vi "setExposureTime.vi"(0 "sCMOS cluster":cluster{"init":i16, "sCMOS handle":u32}, 1 "Exposure time (s)":dbl=0.009997714285714285) -> ()   [LabVIEW 2015]
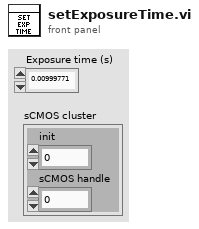
[diagram p1: front panel]
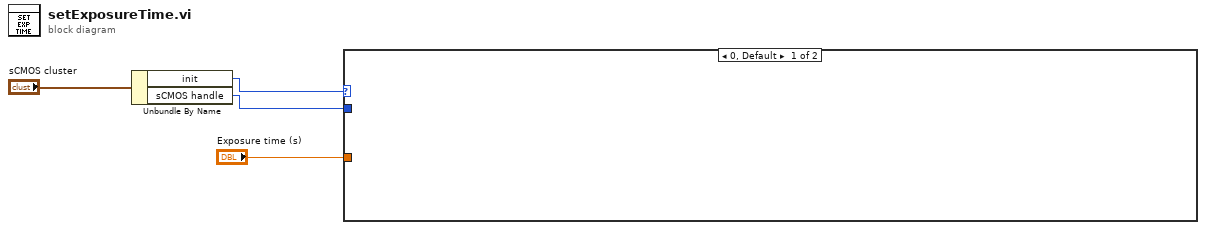
[diagram p0: block diagram]
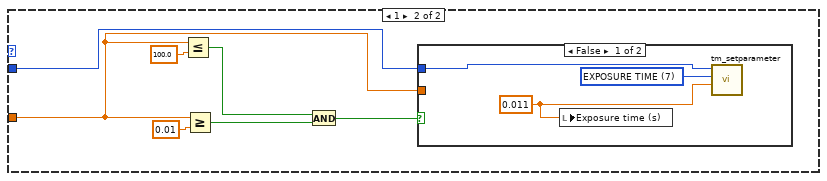
[diagram p2: hidden frame]
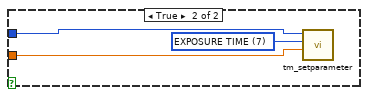
[diagram p3: hidden frame]
diagram:
  n1 = Unbundle By Name("sCMOS cluster") -> ("init"=w3:i16, "sCMOS handle"=w2:u32)
  n2 = case shown="0, Default" w3 {
    tunnel: "Exposure time (s)" -> [_ w5]
    tunnel: w2 -> [_ w11]
    frame 0, Default {
    }
    frame 1 {
      n3 = Less Or Equal?(x=w5, y=100.0 ("x")) -> (x <= y?=w8:bool)
      n4 = Greater Or Equal?(x=w5, y=0.01 ("x")) -> (x >= y?=w10:bool)
      n5 = And(x=w8, y=w10) -> (x .and. y?=w7:bool)
      n6 = case shown="False" w7 {
        tunnel: w11 -> [w14 w17]
        tunnel: w5 -> [_ w16]
        frame False {
          w12 = u32 7 items=["BINNING"=4215968, "BITS PER CHANNEL"=2, "ACTIVE VIEW INDEX"=3, "CCD MODE"=4, "SENSOR MODE"=5, "READOUT MODE"=6, "EXPOSURE TIME"=7, "CONTRAST GAIN"=8, "CONTRAST OFFSET"=9, "LIGHT MODE"=10, "SENSITIVITY"=11, "WHITE BALANCE"=12, "PHOTON IMAGING MODE"=13, "HIGH DYNAMIC RANGE MODE"=14, "TRIGGER SOURCE"=15, "TRIGGER ACTIVE"=16, "TRIGGER MODE"=17, "TRIGGER POLARITY"=18, "TRIGGER GLOBAL EXPOSURE"=19, "FIRST TRIGGER BEHAVIOR"=20, "TRIGGER TIMES"=21, "OUTPUT TRIGGER POLARITY"=22, "OUTPUT TRIGGER DELAY"=23, "OUTPUT TRIGGER PERIOD"=24, "TEMPERATURE"=25, "TEMPERATURE TARGET"=26, "SENSOR COOLER FAN"=27, "MECHANICAL SHUTTER"=28, "BACK FOCUS POSITION"=29, "FRAMEBUNDLE MODE"=30, "FRAMEBUNDLE NUMBER"=31, "LINEBUNDLE HEIGHT"=32, "TRIGGER CONNECTOR"=33, "IMAGE PIXEL TYPE"=34, "OUTPUT TRIGGER KIND"=35, "READOUT DIRECTION"=36, "CHANNEL SYNC"=37] ("Parameter")
          w13 = 0.011 ("Value in")
          n7 = local write "Exposure time (s)"(w13) -> ()
          n8 = call <userlib>:"tm_setparameter.vi"("Value in"=w13, "Parameter"=w12, "Handle in"=w14) -> ()  [unwired: 7 in, 2 out]
        }
        frame True {
          w15 = u32 7 items=["BINNING"=4215968, "BITS PER CHANNEL"=2, "ACTIVE VIEW INDEX"=3, "CCD MODE"=4, "SENSOR MODE"=5, "READOUT MODE"=6, "EXPOSURE TIME"=7, "CONTRAST GAIN"=8, "CONTRAST OFFSET"=9, "LIGHT MODE"=10, "SENSITIVITY"=11, "WHITE BALANCE"=12, "PHOTON IMAGING MODE"=13, "HIGH DYNAMIC RANGE MODE"=14, "TRIGGER SOURCE"=15, "TRIGGER ACTIVE"=16, "TRIGGER MODE"=17, "TRIGGER POLARITY"=18, "TRIGGER GLOBAL EXPOSURE"=19, "FIRST TRIGGER BEHAVIOR"=20, "TRIGGER TIMES"=21, "OUTPUT TRIGGER POLARITY"=22, "OUTPUT TRIGGER DELAY"=23, "OUTPUT TRIGGER PERIOD"=24, "TEMPERATURE"=25, "TEMPERATURE TARGET"=26, "SENSOR COOLER FAN"=27, "MECHANICAL SHUTTER"=28, "BACK FOCUS POSITION"=29, "FRAMEBUNDLE MODE"=30, "FRAMEBUNDLE NUMBER"=31, "LINEBUNDLE HEIGHT"=32, "TRIGGER CONNECTOR"=33, "IMAGE PIXEL TYPE"=34, "OUTPUT TRIGGER KIND"=35, "READOUT DIRECTION"=36, "CHANNEL SYNC"=37] ("Parameter")
          n9 = call <userlib>:"tm_setparameter.vi"("Value in"=w16, "Parameter"=w15, "Handle in"=w17) -> ()  [unwired: 7 in, 2 out]
        }
      }
    }
  }
